vi "Warm Up Measurement.vi"(8 "error in":errorcluster, 10 "timeout (ms)":i32=30000, 11 "gRPC ID":T1) -> (0 "error out":errorcluster, 3 "gRPC ID out":T1)   [LabVIEW 2021, in "MeasurementServerTests.lvlib" / "Measurement Service Tests.lvlib" / "Continuous Counting Client.lvlib"]
uses:
  Continuous Counting Client.lvlib
  <vilib>/gRPC/LabVIEW gRPC Library/Shared/grpcId.ctl
  gRPC/Generated APIs/ni/measurementlink/measurement/v2/Measurement Service Client V2/Measurement Service Client V2.lvlib
  <vilib>/gRPC/LabVIEW gRPC Library/grpc-lvsupport-release.lvlib
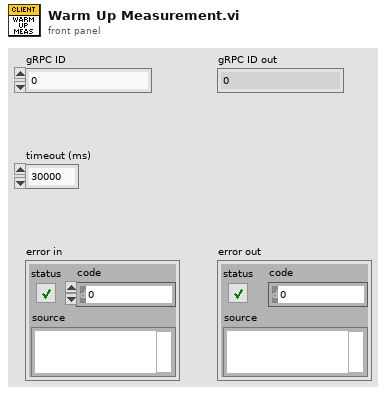
[diagram p1: front panel]
types:
  T1 = typedef "grpc-lvsupport-release.lvlib/grpcId.ctl" = u64
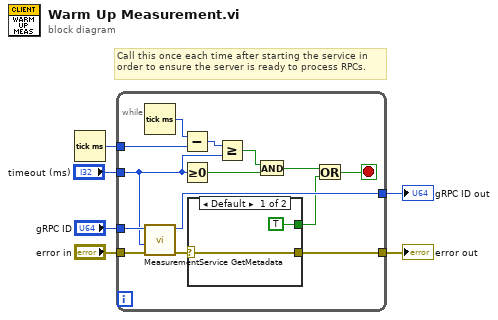
[diagram p0: block diagram]
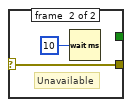
[diagram p2: hidden frame]
diagram:
  # "Call this once each time after starting the service in\norder to ensure the server is ready to process RPCs."
  n1 = Tick Count (ms)() -> (millisecond timer value=w1:u32)
  n2 = while {
    tunnel: [w20] -> w3
    tunnel: "error in" -> [w19]
    tunnel: "timeout (ms)" -> [w11]
    tunnel: "gRPC ID" -> [w18]
    tunnel: [w17] -> w4
    tunnel: w1 -> [w13]
    stop <- w7 stop-if-true
    n3 = Tick Count (ms)() -> (millisecond timer value=w14:u32)
    n4 = call "MeasurementService GetMetadata.vi"("error in"=w19, "timeout (ms)"=w11, "gRPC ID"=w18) -> ("error out"=w16:errorcluster, "gRPC ID out"=w17:T1)  [unwired: 6 in, 1 out]
    n5 = Subtract(x=w14, y=w13) -> (x-y=w12:u32)
    n6 = Greater Or Equal To 0?(x=w11) -> (x >= 0?=w9:bool)
    n7 = case shown="Default" w16 {
      selector: w16 -> [w22 w24]
      tunnel: [w22 w24] -> w20
      tunnel: [TRUE _] -> w15
      frame #0 {
      }
      frame #1 {
        # "Unavailable"
        n8 = Wait (ms)(milliseconds to wait=u32 10) -> ()  [unwired: 1 out]
      }
    }
    n9 = Greater Or Equal?(x=w12, y=w11) -> (x >= y?=w10:bool)
    n10 = And(x=w10, y=w9) -> (x .and. y?=w8:bool)
    n11 = Or(x=w8, y=w15) -> (x .or. y?=w7:bool)
  }
  "gRPC ID out" <- w4
  "error out" <- w3
